vi "2 MissionSetpoints.vi"() -> (2 "Setpoints Out":T1)   [LabVIEW 2011]
doc: "The MissionSetpoints VI determines the best sail and rudder setpoints to get to the current goal. Currently it implements a simple system based off of a series of waypoints that points the bow of the ship in the direction of the next waypoint."
uses:
  2 Typedefs/setpoints to arbiter.ctl
panel:
  out "Optimal Heading":dbl
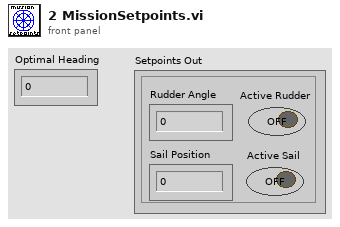
[diagram p1: front panel]
types:
  T1 = typedef "setpoints to arbiter.ctl" = cluster{"Rudder Angle":dbl, "Sail Position":dbl, "Active Rudder":bool, "Active Sail":bool}
  T2 = typedef "sail setpt.ctl" = dbl
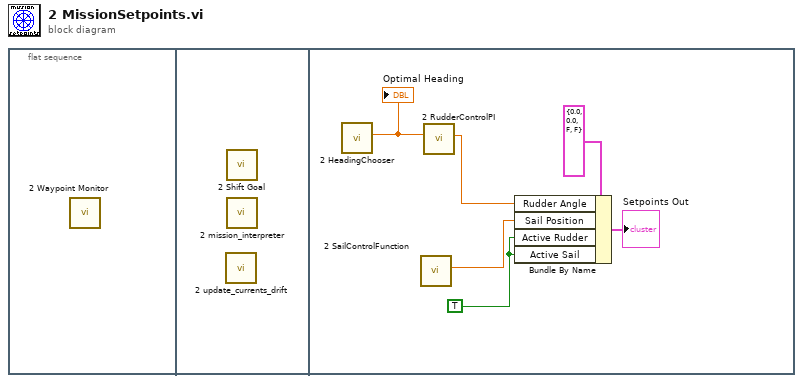
[diagram p0: block diagram]
diagram:
  n1 = flat-sequence {
    frame #0 {
      n2 = call "2 Waypoint Monitor.vi"() -> ()  [unwired: 12 in]
    }
    frame #1 {
      n3 = call "2 update_currents_drift.vi"() -> ()  [unwired: 12 in]
      n4 = call "2 Shift Goal.vi"() -> ()  [unwired: 12 in]
      n5 = call "2 mission_interpreter.vi"() -> ()  [unwired: 11 in, 1 out]
    }
    frame #2 {
      w3 = TRUE
      n6 = call "2 HeadingChooser.vi"() -> ("Optimal Heading"=w1:dbl)  [unwired: 9 in, 2 out]
      "Optimal Heading" <- w1
      n7 = call "2 SailControlFunction.vi"() -> ("Sail Position"=w4:T2)  [unwired: 11 in]
      n8 = call "2 RudderControlPI.vi"("Desired Heading"=w1) -> ("Rudder Output"=w2:dbl)  [unwired: 10 in]
      n9 = Bundle By Name(cluster=T1 {"Rudder Angle"=0.0, "Sail Position"=0.0, "Active Rudder"=FALSE, "Active Sail"=FALSE} ("Setpoints Out"), "Rudder Angle"=w2, "Sail Position"=w4, "Active Rudder"=w3, "Active Sail"=w3) -> (→"Setpoints Out":T1)
    }
  }
